vi "FlipArray.vi"(11 "In":dbl[][](array[numeric])) -> (3 "Out":dbl[][](array[numeric]))   [LabVIEW 2020]
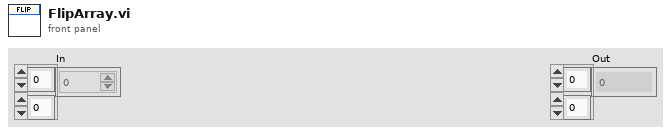
[diagram p1: front panel]
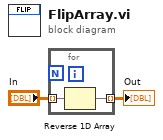
[diagram p0: block diagram]
diagram:
  n1 = for {
    tunnel: "In" -> [w4] mode=indexing
    tunnel: [w3] -> w1 mode=indexing
    n2 = Reverse 1D Array(array=w4) -> (reversed array=w3:dbl[])
  }
  "Out" <- w1
